vi "Test Get Failed Items after Consecutive Tests.vi"(8 "error in (no error)":errorcluster, 11 "Result Model Result Recording Test in":refnum<class "Result Model Result Recording Test.lvclass">) -> (0 "error out":errorcluster, 3 "Result Model Result Recording Test out":refnum<class "Result Model Result Recording Test.lvclass">)   [LabVIEW 2020, in "Result Model Result Recording Test.lvclass"]
uses:
  Result Model Result Recording Test.lvclass
  C:/Program Files (x86)/National Instruments/LabVIEW 2020/vi.lib/Astemes/LUnit/Test Case.lvclass
  source/Core/Result/Result.ctl
  source/Core/Result/Status.ctl
  source/Core/Result/Type.ctl
  source/User Interface/Result Model/Tree Item Filter.ctl
  <vilib>/Astemes/LUnit/Test Case.lvclass/Test Case.ctl
  ae2c71b8-32bb-49d1-8500-0119bfec74ff.vi
  <vilib>/Astemes/LUnit/Append Pass Result.vi
  <vilib>/Astemes/LUnit/Append Fail Result.vi
  <vilib>/Astemes/LUnit/Compare Variants.vi
  <vilib>/Astemes/LUnit/Describe Comparison.vi
  <vilib>/Astemes/LUnit/Variant to string.vi
  <vilib>/Utility/Data Type/Get Type Information.vi
  <vilib>/Utility/LVClass/Get LV Class Name.vi
  source/User Interface/Result Model/Result Model.lvclass
  source/Core/Result/Result.lvlib
panel:
  out "Tree Items":T1(array[cluster])
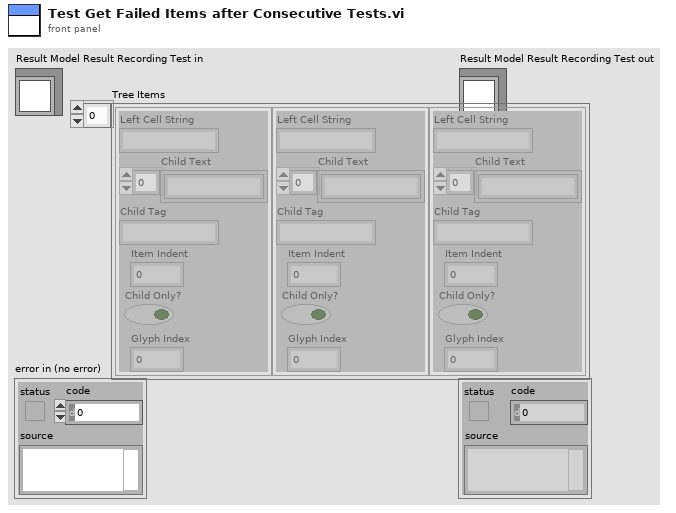
[diagram p1: front panel]
types:
  T1 = cluster{"Left Cell String":string, "Child Text":string[], "Child Tag":string, "Item Indent":i32, "Child Only?":bool, "Glyph Index":i32}[]
  T2 = typedef "Result Model.lvclass/Tree Item Filter.ctl" = enum16{"All", "Only Fails"}
  T3 = typedef "Result.lvlib/Result.ctl" = cluster{"Name":string, "Message":string, "Description":string, "Status":T4, "Result Type":T5, "Execution Time":dbl}
  T4 = typedef "Result.lvlib/Status.ctl" = enum16{"", "Passed", "Failed", "Error", "Skipped", "Setup Error", "Broken", "Teardown Error"}
  T5 = typedef "Result.lvlib/Type.ctl" = enum16{"Test Case", "Test Suite", "Test Run", "Pass", "Fail", "Skip", "Pass if", "Fail if", "Pass if Error", "Fail if Error", "Pass if Equal", "Fail if Equal"}
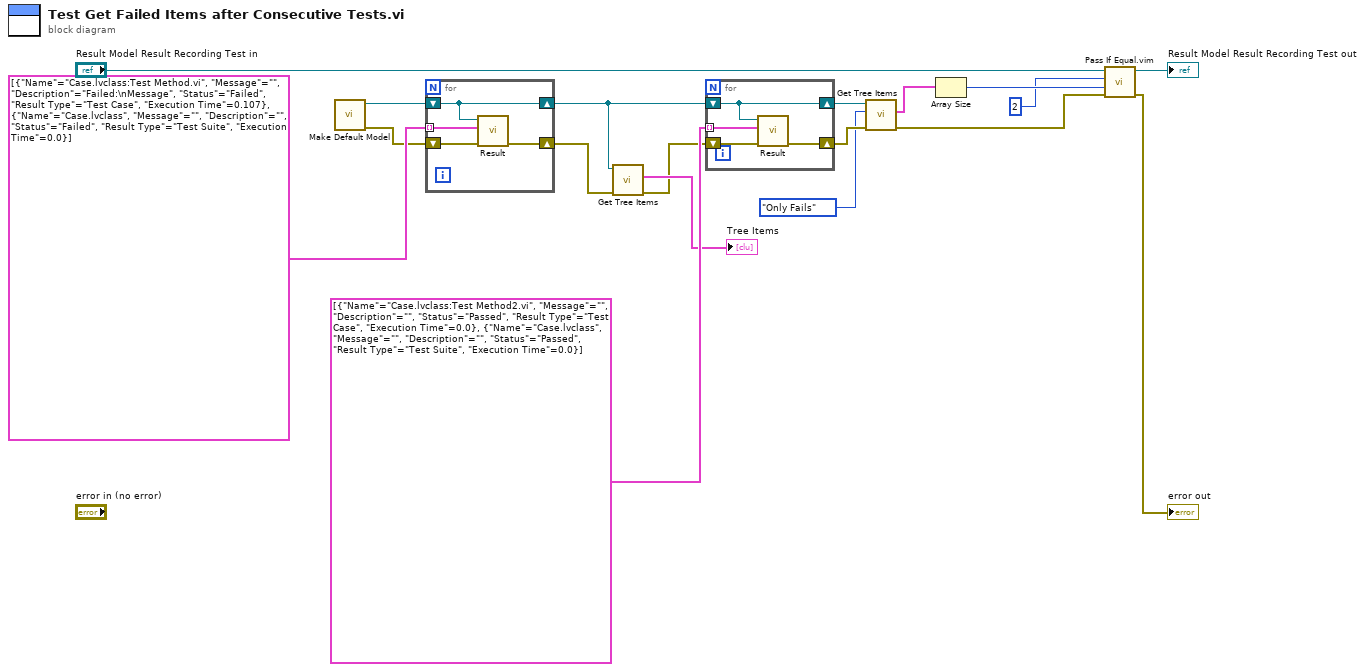
[diagram p0: block diagram]
diagram:
  n1 = call "Make Default Model.vi"() -> ("error out"=w11:errorcluster, "Result Model out"=w18:refnum<class "Result Model.lvclass">)  [unwired: 10 in]
  n2 = for {
    tunnel: T3[] [{"Name"="Case.lvclass:Test Method.vi", "Message"="", "Description"="Failed:\nMessage", "Status"=enum."Failed", "Result Type"=enum."Test Case", "Execution Time"=0.107}, {"Name"="Case.lvclass", "Message"="", "Description"="", "Status"=enum."Failed", "Result Type"=enum."Test Suite", "Execution Time"=0.0}] ("Results") -> [w22] mode=indexing
    shift-right: [w21] -> w4
    shift-left: w18 -> [w21]
    shift-right: [w20] -> w2
    shift-left: w11 -> [w19]
    n3 = call-dynamic "Result.vi"("error in (no error)"=w19, "Results"=w22, "Result Model in"=w21) -> ("error out"=w20:errorcluster)  [unwired: 8 in]
  }
  n4 = call "Get Tree Items.vi"("error in (no error)"=w2, "Result Model In"=w4) -> ("error out"=w1:errorcluster, "Tree Items"=→"Tree Items":T1)  [unwired: 8 in]
  n5 = for {
    tunnel: T3[] [{"Name"="Case.lvclass:Test Method2.vi", "Message"="", "Description"="", "Status"=enum."Passed", "Result Type"=enum."Test Case", "Execution Time"=0.0}, {"Name"="Case.lvclass", "Message"="", "Description"="", "Status"=enum."Passed", "Result Type"=enum."Test Suite", "Execution Time"=0.0}] ("Results") -> [w26] mode=indexing
    shift-right: [w25] -> w9
    shift-left: w4 -> [w25]
    shift-right: [w23] -> w8
    shift-left: w1 -> [w24]
    n6 = call-dynamic "Result.vi"("error in (no error)"=w24, "Results"=w26, "Result Model in"=w25) -> ("error out"=w23:errorcluster)  [unwired: 8 in]
  }
  n7 = call "Get Tree Items.vi"("error in (no error)"=w8, "Filter"=Tree_Item_Filter."Only Fails", "Result Model In"=w9) -> ("error out"=w5:errorcluster, "Tree Items"=w6:T1)  [unwired: 7 in]
  n8 = Array Size(array=w6) -> (size(s)=w13:i32)
  n9 = call "Pass If Equal.vim"("error in (no error)"=w5, "Actual"=w13, "Expected"=2 ("size(s)"), "LUnit Test Case In"="Result Model Result Recording Test in") -> ("error out"=→"error out":errorcluster, "LUnit Test Case Out"=→"Result Model Result Recording Test out":refnum<class "Result Model Result Recording Test.lvclass">)  [unwired: 6 in]
